vi "getDeviceInfo.vi"(8 "error in":errorcluster, 11 "connection ID in":refnum<k5>) -> (0 "error out":errorcluster, 2 "device info":T1, 3 "connection ID":refnum<k5>)   [LabVIEW 2016]
panel:
  in  "Cluster":T2
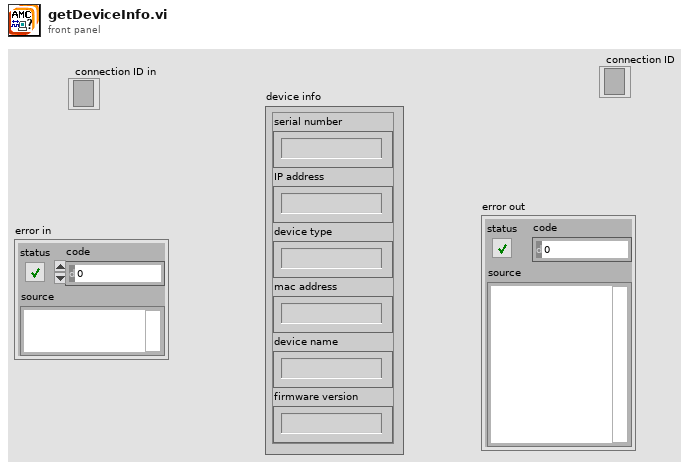
[diagram p1: front panel]
types:
  T1 = cluster{"serial number":string, "IP address":string, "device type":string, "mac address":string, "device name":string, "firmware version":string}
  T2 = cluster{"Serial":string, "IP Address":string, "devicetype":string, "macAddress":string, "deviceName":string, "Firmware Version":string}
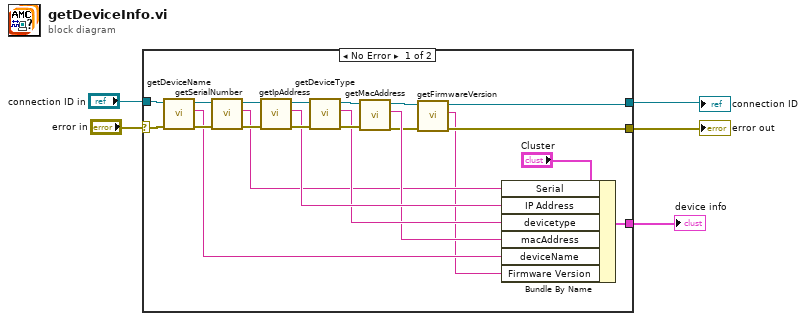
[diagram p0: block diagram]
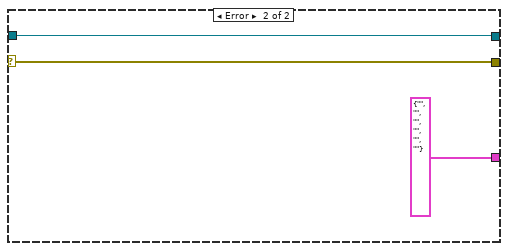
[diagram p2: hidden frame]
diagram:
  n1 = case shown="No Error" "error in" {
    selector: "error in" -> [w12 w29]
    tunnel: "connection ID in" -> [w15 w30]
    tunnel: [w8 w30] -> w4
    tunnel: [w9 w29] -> w3
    tunnel: [w7 T2 {"Serial"="", "IP Address"="", "devicetype"="", "macAddress"="", "deviceName"="", "Firmware Version"=""} ("Cluster 2")] -> w1
    frame No Error {
      n2 = call "getDeviceName.vi"("error in"=w12, "connection ID"=w15) -> ("error out"=w24:errorcluster, "string"=w13:string, "connection ID"=w27:refnum<k5>)  [unwired: 7 in]
      n3 = call "getSerialNumber.vi"("error in"=w24, "connection ID"=w27) -> ("error out"=w25:errorcluster, "string"=w14:string, "connection ID"=w26:refnum<k5>)  [unwired: 7 in]
      n4 = call "getIpAddress.vi"("error in"=w25, "connection ID"=w26) -> ("error out"=w23:errorcluster, "IP"=w18:string, "connection ID"=w22:refnum<k5>)  [unwired: 7 in]
      n5 = call "getDeviceType.vi"("error in"=w23, "connection ID"=w22) -> ("error out"=w20:errorcluster, "devicetype"=w17:string, "connection ID"=w21:refnum<k5>)  [unwired: 7 in]
      n6 = call "getMacAddress.vi"("error in"=w20, "connection ID"=w21) -> ("error out"=w10:errorcluster, "string"=w16:string, "connection ID"=w11:refnum<k5>)  [unwired: 7 in]
      n7 = call "getFirmwareVersion.vi"("error in"=w10, "connection ID"=w11) -> ("error out"=w9:errorcluster, "string"=w6:string, "connection ID"=w8:refnum<k5>)  [unwired: 7 in]
      n8 = Bundle By Name(cluster="Cluster", "Serial"=w14, "IP Address"=w18, "devicetype"=w17, "macAddress"=w16, "deviceName"=w13, "Firmware Version"=w6) -> (w7:T2)
    }
    frame Error {
    }
  }
  "connection ID" <- w4
  "error out" <- w3
  "device info" <- w1
